vi "CulverDrive.vi"(8 "quick turn":bool, 9 "Wheel.X":dbl(slide) scale=-1.0..1.0, 10 "Wheel.Y":dbl(slide) scale=-1.0..1.0, 11 "Throttle":dbl(slide) scale=-1.0..1.0) -> (2 "Right Side":dbl(slide) scale=-1.0..1.0, 3 "Left Side":dbl(slide) scale=-1.0..1.0, 5 "Theta":dbl(knob) scale=-180.0..180.0, 7 "R":dbl(knob) scale=0.0..1.0)   [LabVIEW 2017]
panel:
  in  "radius_curve":dbl[](array[numeric])=[1.0, 1.0, 0.0, 0.0, 0.0]
  in  "raw_curve":dbl[](array[numeric])=[0.0, 0.0, 1.0, 1.0, 0.0]
  in  "theta_axis":dbl[](array[numeric])=[0.0, 95.0, 115.0, 170.0, 180.0]
  in  "radius gain":dbl=1.2
  in  "raw gain":dbl=1.4
  out "Forward Component":dbl(slide) scale=0.0..1.0
  out "Raw Component":dbl(slide) scale=0.0..1.0
  out "Radius Component":dbl(slide) scale=0.0..1.0
  out "Raw":dbl(slide) scale=0.0..1.0
  out "Radius":dbl(slide) scale=0.0..1.0
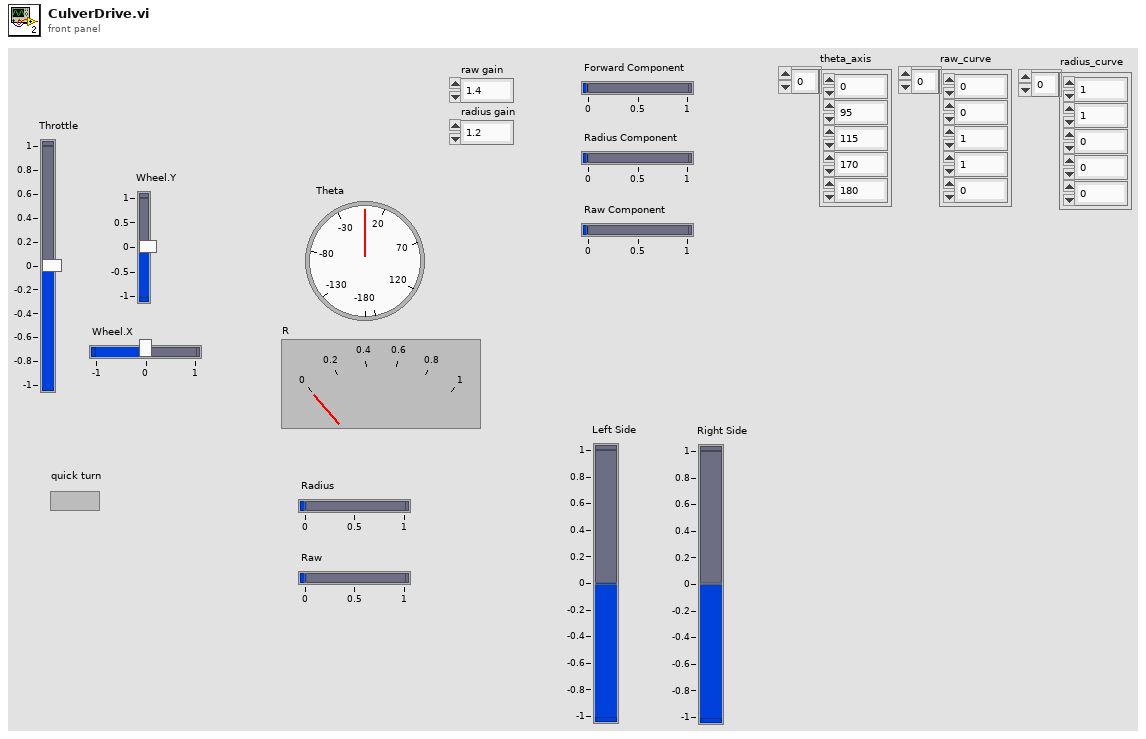
[diagram p1: front panel]
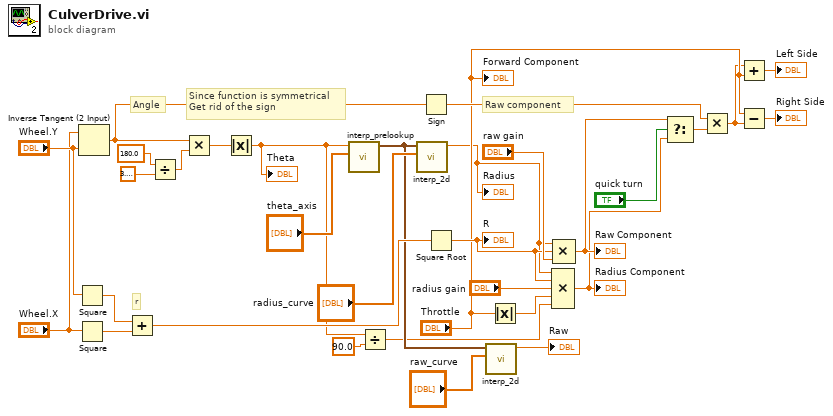
[diagram p0: block diagram]
diagram:
  # "r"
  # "Raw component"
  # "Since function is symmetrical\nGet rid of the sign"
  # "Angle"
  n1 = Square(x="Wheel.Y") -> (x^2=w25:dbl)
  n2 = Square(x="Wheel.X") -> (x^2=w24:dbl)
  n3 = Inverse Tangent (2 Input)(1:"Wheel.Y", 2:"Wheel.X") -> (0:w28:dbl)
  n4 = Add(x=w25, y=w24) -> (x+y=w23:dbl)
  n5 = Divide(x=180.0, y=3.141592653589793) -> (x/y=w30:dbl)
  n6 = Multiply(x=w28, y=w30) -> (x*y=w29:dbl)
  n7 = Absolute Value(x=w29) -> (abs(x)=w12:dbl)
  "Theta" <- w12
  n8 = call "interp_prelookup.vi"("x"="theta_axis", "X"=w12) -> ("prelookup"=w13:cluster{"frac":dbl, "num":u8})  [unwired: 8 in, 1 out]
  n9 = Divide(x=w12, y=90.0) -> (x/y=w10:dbl)
  n10 = call "interp_2d.vi"("z"="radius_curve", "prelookup"=w13) -> ("z"=w1:dbl)  [unwired: 9 in]
  "Radius" <- w1
  n11 = Sign(1:w28) -> (0:w20:dbl)
  n12 = Square Root(x=w23) -> (sqrt(x)=w9:dbl)
  "R" <- w9
  n13 = call "interp_2d.vi"("z"="raw_curve", "prelookup"=w13) -> ("z"=→"Raw":dbl)  [unwired: 9 in]
  n14 = Absolute Value(x="Throttle") -> (abs(x)=w8:dbl)
  n15 = Compound Arithmetic op=MULTIPLY(w1, w9, "radius gain", w8, w10) -> (w3:dbl)
  "Radius Component" <- w3
  n16 = Compound Arithmetic op=MULTIPLY(w1, w9, "raw gain") -> (w4:dbl)
  "Raw Component" <- w4
  n17 = Select(t=w4, s="quick turn", f=w3) -> (s? t:f=w5:dbl)
  n18 = Multiply(x=w20, y=w5) -> (x*y=w6:dbl)
  n19 = Add(x=w6, y="Throttle") -> (x+y=→"Left Side":dbl)
  n20 = Subtract(x="Throttle", y=w6) -> (x-y=→"Right Side":dbl)
  "Forward Component" <- "Throttle"
